vi "Shift Registers.vi"() -> ()   [LabVIEW 2020]
panel:
  out "Output":i32
  out "Iterations":i32
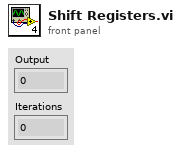
[diagram p1: front panel]
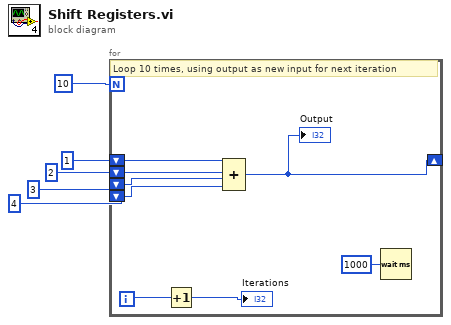
[diagram p0: block diagram]
diagram:
  n1 = for {
    N: 10 -> [_]
    shift-right: [w6] -> _
    shift-left: 1 ("x") -> [w10]
    shift-left: 2 ("x") -> [w9]
    shift-left: 3 ("x") -> [w8]
    shift-left: 4 ("x") -> [w7]
    i -> [w12]
    # "Loop 10 times, using output as new input for next iteration"
    n2 = Increment(x=w12) -> (x+1=→"Iterations":i32)
    n3 = Compound Arithmetic op=ADD(w10, w9, w8, w7) -> (w6:i32)
    "Output" <- w6
    n4 = Wait (ms)(milliseconds to wait=u32 1000) -> ()  [unwired: 1 out]
  }
